vi "Read.vi"(8 "error in (no error)":errorcluster, 9 "timeout ms":i32, 11 "Connection Data":T1) -> (0 "error out":errorcluster, 3 "Connection Data out":T1)   [LabVIEW 2014, in "FrontPanelPublisher.lvlib" / "Websocket.lvclass"]
uses:
  Websocket.lvclass
  ConnectionData.ctl
  FrontPanelManager_class/FrontPanelManager.lvclass
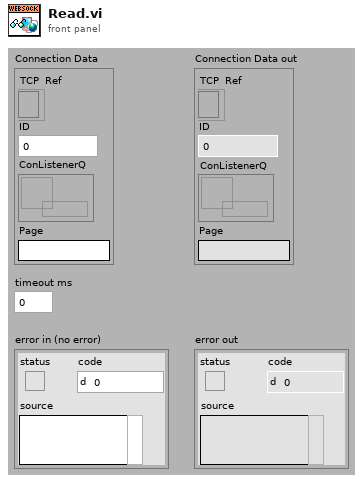
[diagram p1: front panel]
types:
  T1 = typedef "FrontPanelPublisher.lvlib/Websocket.lvclass/ConnectionData.ctl" = cluster{"TCP  Ref":refnum<k5>, "connection ID":u64, "ConListenerQ":refnum<queue>, "Page":string}
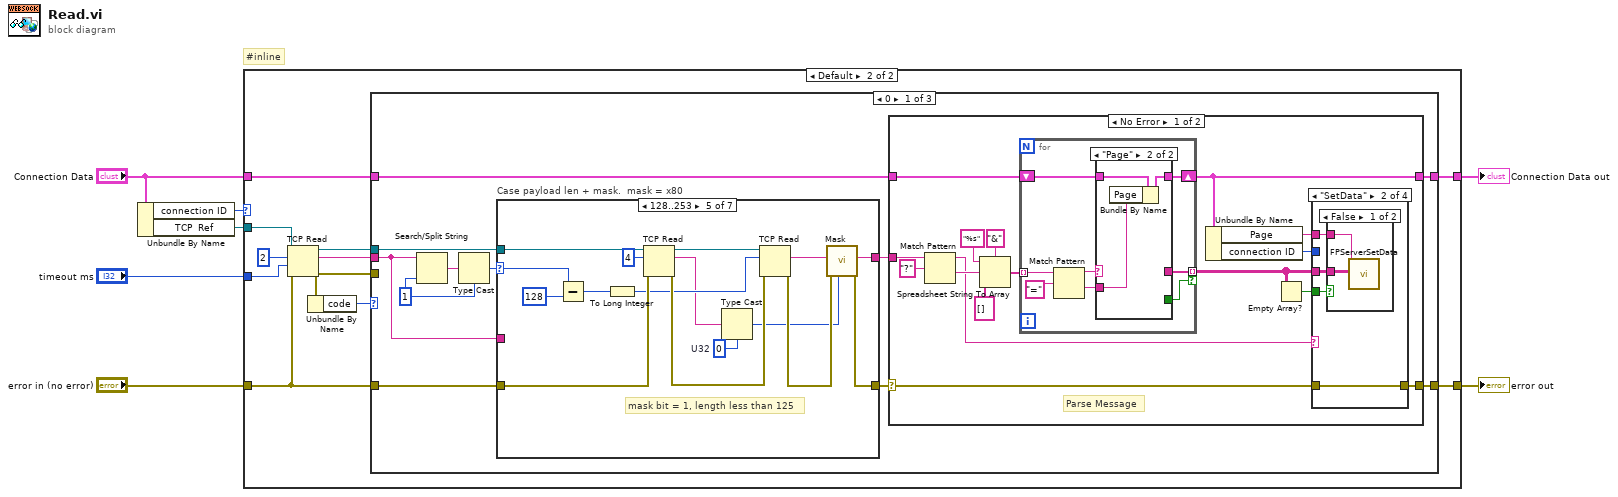
[diagram p0: block diagram]
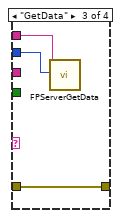
[diagram p5: hidden frame]
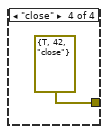
[diagram p6: hidden frame]
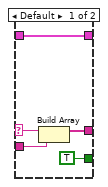
[diagram p7: hidden frame]
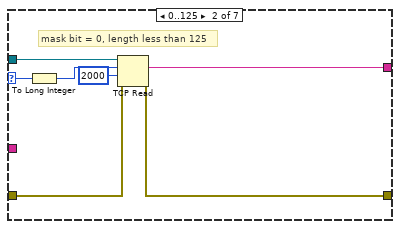
[diagram p10: hidden frame]
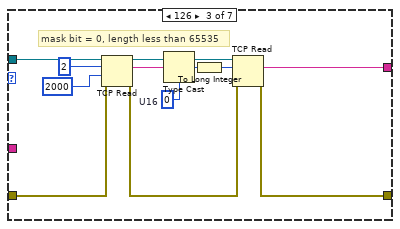
[diagram p11: hidden frame]
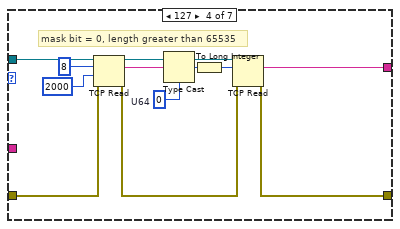
[diagram p12: hidden frame]
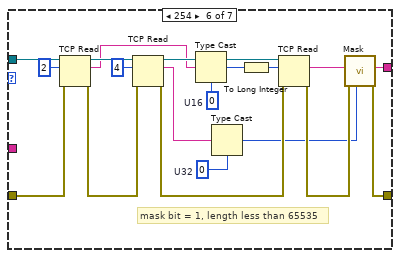
[diagram p13: hidden frame]
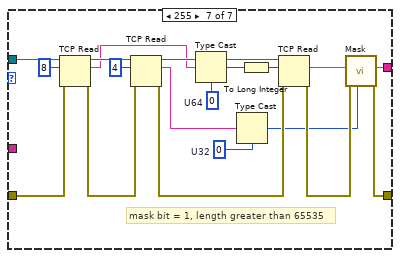
[diagram p14: hidden frame]
diagram:
  # "#inline"
  n1 = Unbundle By Name("Connection Data") -> ("connection ID"=w2:u64, "TCP  Ref"=w5:refnum<k5>)
  n2 = case shown="Default" w2 {
    tunnel: "timeout ms" -> [_ w20]
    tunnel: "error in (no error)" -> [w9 w16]
    tunnel: w5 -> [_ w15]
    tunnel: "Connection Data" -> [w8 w12]
    tunnel: [w9 w11] -> w3
    tunnel: [w8 w10] -> w1
    frame 0 {
    }
    frame Default {
      n3 = TCP Read(connection ID=w15, bytes to read=2, error in (no error)=w16, 9:w20) -> (connection ID out=w17:refnum<k5>, data out=w19:string, error out=w14:errorcluster)  [unwired: 1 in]
      n4 = Unbundle By Name(w14) -> ("code"=w13:i32)
      n5 = case shown="0" w13 {
        tunnel: w19 -> [w27 _ _]
        tunnel: w17 -> [w26 _ _]
        tunnel: [w22 w164 w166] -> w11
        tunnel: w16 -> [w31 w164 _]
        tunnel: w14 -> [_ _ w166]
        tunnel: w12 -> [w23 w163 w165]
        tunnel: [w21 w163 w165] -> w10
        frame 0 {
          w29 = u8 1 ("offset (0)")
          n6 = Search/Split String(string=w27, offset (0)=w29) -> (match + rest of string=w30:string)  [unwired: 1 in, 2 out]
          n7 = Type Cast(type=w29, x=w30) -> (*(type *) &x=w28:u8)
          n8 = case "Case payload len + mask.  mask = x80" shown="128..253" w28 {
            selector: w28 -> [_ w81 _ _ w119 _ _]
            tunnel: [_ w78 w85 w97 w112 w128 w147] -> w24
            tunnel: w27 -> [_ _ _ _ _ _ _]
            tunnel: w26 -> [_ w82 w93 w105 w120 w138 w157]
            tunnel: [w77 w84 w95 w107 w122 w140 w159] -> w25
            tunnel: w31 -> [w77 w83 w94 w106 w121 w139 w158]
            frame Default {
              # "error"
            }
            frame 0..125 {
              # "mask bit = 0, length less than 125"
              n9 = To Long Integer(number=w81) -> (32bit integer=w79:i32)
              n10 = TCP Read(connection ID=w82, bytes to read=w79, error in (no error)=w83, 9:2000 ("timeout ms (25000)")) -> (data out=w78:string, error out=w84:errorcluster)  [unwired: 1 in, 1 out]
            }
            frame 126 {
              w87 = u16 0  # U16
              # "mask bit = 0, length less than 65535"
              n11 = TCP Read(connection ID=w93, bytes to read=2, error in (no error)=w94, 9:2000 ("timeout ms (25000)")) -> (connection ID out=w90:refnum<k5>, data out=w89:string, error out=w96:errorcluster)  [unwired: 1 in]
              n12 = Type Cast(type=w87, x=w89) -> (*(type *) &x=w88:u16)
              n13 = To Long Integer(number=w88) -> (32bit integer=w86:i32)
              n14 = TCP Read(connection ID=w90, bytes to read=w86, error in (no error)=w96) -> (data out=w85:string, error out=w95:errorcluster)  [unwired: 2 in, 1 out]
            }
            frame 127 {
              w99 = u64 0  # U64
              # "mask bit = 0, length greater than 65535"
              n15 = TCP Read(connection ID=w105, bytes to read=8, error in (no error)=w106, 9:2000 ("timeout ms (25000)")) -> (connection ID out=w102:refnum<k5>, data out=w101:string, error out=w108:errorcluster)  [unwired: 1 in]
              n16 = Type Cast(type=w99, x=w101) -> (*(type *) &x=w100:u64)
              n17 = To Long Integer(number=w100) -> (32bit integer=w98:i32)
              n18 = TCP Read(connection ID=w102, bytes to read=w98, error in (no error)=w108) -> (data out=w97:string, error out=w107:errorcluster)  [unwired: 2 in, 1 out]
            }
            frame 128..253 {
              w110 = u32 0  # U32
              # "mask bit = 1, length less than 125"
              n19 = Subtract(x=w119, y=u8 128) -> (x-y=w115:u8)
              n20 = To Long Integer(number=w115) -> (32bit integer=w114:i32)
              n21 = TCP Read(connection ID=w120, bytes to read=4, error in (no error)=w121) -> (connection ID out=w116:refnum<k5>, data out=w111:string, error out=w124:errorcluster)  [unwired: 2 in]
              n22 = Type Cast(type=w110, x=w111) -> (*(type *) &x=w109:u32)
              n23 = TCP Read(connection ID=w116, bytes to read=w114, error in (no error)=w124) -> (data out=w113:string, error out=w123:errorcluster)  [unwired: 2 in, 1 out]
              n24 = call "Mask.vi"("mask key"=w109, "error in (no error)"=w123, "mask/unmask string in"=w113) -> ("error out"=w122:errorcluster, "mask/unmask string out"=w112:string)  [unwired: 5 in]
            }
            frame 254 {
              w126 = u32 0  # U32
              w133 = u16 0  # U16
              # "mask bit = 1, length less than 65535"
              n25 = TCP Read(connection ID=w138, bytes to read=2, error in (no error)=w139) -> (connection ID out=w136:refnum<k5>, data out=w130:string, error out=w143:errorcluster)  [unwired: 2 in]
              n26 = TCP Read(connection ID=w136, bytes to read=4, error in (no error)=w143) -> (connection ID out=w132:refnum<k5>, data out=w127:string, error out=w142:errorcluster)  [unwired: 2 in]
              n27 = Type Cast(type=w133, x=w130) -> (*(type *) &x=w134:u16)
              n28 = Type Cast(type=w126, x=w127) -> (*(type *) &x=w125:u32)
              n29 = To Long Integer(number=w134) -> (32bit integer=w131:i32)
              n30 = TCP Read(connection ID=w132, bytes to read=w131, error in (no error)=w142) -> (data out=w129:string, error out=w141:errorcluster)  [unwired: 2 in, 1 out]
              n31 = call "Mask.vi"("mask key"=w125, "error in (no error)"=w141, "mask/unmask string in"=w129) -> ("error out"=w140:errorcluster, "mask/unmask string out"=w128:string)  [unwired: 5 in]
            }
            frame 255 {
              w145 = u32 0  # U32
              w152 = u64 0  # U64
              # "mask bit = 1, length greater than 65535"
              n32 = TCP Read(connection ID=w157, bytes to read=8, error in (no error)=w158) -> (connection ID out=w155:refnum<k5>, data out=w149:string, error out=w162:errorcluster)  [unwired: 2 in]
              n33 = TCP Read(connection ID=w155, bytes to read=4, error in (no error)=w162) -> (connection ID out=w151:refnum<k5>, data out=w146:string, error out=w161:errorcluster)  [unwired: 2 in]
              n34 = Type Cast(type=w152, x=w149) -> (*(type *) &x=w153:u64)
              n35 = Type Cast(type=w145, x=w146) -> (*(type *) &x=w144:u32)
              n36 = To Long Integer(number=w153) -> (32bit integer=w150:i32)
              n37 = TCP Read(connection ID=w151, bytes to read=w150, error in (no error)=w161) -> (data out=w148:string, error out=w160:errorcluster)  [unwired: 2 in, 1 out]
              n38 = call "Mask.vi"("mask key"=w144, "error in (no error)"=w160, "mask/unmask string in"=w148) -> ("error out"=w159:errorcluster, "mask/unmask string out"=w147:string)  [unwired: 5 in]
            }
          }
          n39 = case shown="No Error" w25 {
            selector: w25 -> [w33 w76]
            tunnel: [w34 w76] -> w22
            tunnel: w24 -> [w38 _]
            tunnel: w23 -> [w47 w75]
            tunnel: [w32 w75] -> w21
            frame No Error {
              # "Parse Message"
              n40 = Match Pattern(string=w38, regular expression="?") -> (before substring=w36:string, after substring=w37:string)  [unwired: 1 in, 2 out]
              n41 = Spreadsheet String To Array(delimiter (Tab)="&", format string="%s", spreadsheet string=w37, array type (2D Dbl)=string[] []) -> (array=w42:string[])
              n42 = for {
                shift-right: [w63] -> w32
                shift-left: w47 -> [w64]
                tunnel: w42 -> [w61] mode=indexing
                tunnel: [w60] -> w41 mode=indexing if=w59
                n43 = Match Pattern(string=w61, regular expression="=") -> (before substring=w65:string, after substring=w62:string)  [unwired: 1 in, 2 out]
                n44 = case shown="\"Page\"" w65 {
                  selector: w65 -> [w69 _]
                  tunnel: w64 -> [w71 w74]
                  tunnel: [w71 w73] -> w63
                  tunnel: w62 -> [w68 w72]
                  tunnel: [TRUE _] -> w59
                  tunnel: [w67 _] -> w60
                  frame Default {
                    n45 = Build Array(w69, w68) -> (w67:string[])
                  }
                  frame "Page" {
                    n46 = Bundle By Name(cluster=w74, "Page"=w72) -> (w73:T1)
                  }
                }
              }
              n47 = Unbundle By Name(w32) -> ("Page"=w40:string, "connection ID"=w35:u64)
              n48 = Empty Array?(array=w41) -> (empty?=w46:bool)
              n49 = case shown="\"SetData\"" w36 {
                tunnel: w46 -> [_ w52 _ _]
                tunnel: w41 -> [_ w51 _ _]
                tunnel: w40 -> [_ w50 w57 _]
                tunnel: w35 -> [_ _ w56 _]
                tunnel: [w48 w49 w55 errorcluster {"status"=TRUE, "code"=42, "source"="close"} ("error IO")] -> w34
                tunnel: w33 -> [w48 w49 w55 _]
                frame Default {
                }
                frame "SetData" {
                  n50 = case shown="False" w52 {
                    tunnel: w51 -> [w53 _]
                    tunnel: w50 -> [w54 _]
                    frame False {
                      n51 = call "FPServerSetData.vi"("Page"=w54, "Data"=w53) -> ()  [unwired: 17 in, 1 out]
                    }
                    frame True {
                    }
                  }
                }
                frame "GetData" {
                  n52 = call "FPServerGetData.vi"("Page"=w57, "Connection ID"=w56) -> ()  [unwired: 17 in, 1 out]
                }
                frame "close" {
                }
              }
            }
            frame Error {
            }
          }
        }
        frame 56 {
        }
        frame Default {
        }
      }
    }
  }
  "error out" <- w3
  "Connection Data out" <- w1
